vi "Conv2D(CuLab).vi"() -> ()   [LabVIEW 2020]
uses:
  07a04de9-0afa-4073-98d7-d7a9b3666a97.vi
  85e02f6e-3771-4ab4-8b07-b5403419ee50.vi
  <vilib>/Analysis/baseanly.llb/Mean (DBL).vi
  <vilib>/Utility/High Resolution Relative Seconds.vi
  <vilib>/Ngene/CuLab - GPU Accelerated Toolkit/Toolkit/Low_Level/Tensor_Classes/T_Children/T2D/T2D_Children/T2D_SGL/Create_Push.vi
  <vilib>/Ngene/CuLab - GPU Accelerated Toolkit/Toolkit/Low_Level/Tensor_Classes/T_Children/T2D/T2D_Children/T2D_SGL/Create.vi
  <vilib>/Ngene/CuLab - GPU Accelerated Toolkit/Toolkit/Low_Level/Tensor_Classes/T_Children/T2D/T2D_Children/T2D_SGL/Push.vi
  <vilib>/Ngene/CuLab - GPU Accelerated Toolkit/Toolkit/API/Signal Processing/Signal Operation/Convolution/T2D/CU_Convolution_T2D_SGL.vi
  <vilib>/Ngene/CuLab - GPU Accelerated Toolkit/Toolkit/Low_Level/Tensor_Classes/T_Children/T2D/T2D_Children/T2D_SGL/Pull.vi
  <vilib>/Utility/file.llb/Write Delimited Spreadsheet (DBL).vi
  <vilib>/Ngene/CuLab - GPU Accelerated Toolkit/Toolkit/CuLab.lvlib
  <vilib>/Analysis/NI_AALBase.lvlib
  <vilib>/Ngene/CuLab - GPU Accelerated Toolkit/Toolkit/Low_Level/Tensor_Classes/T_Children/T2D/T2D_Children/T2D_SGL/T2D_SGL.lvclass
panel:
  out "Results(s)":dbl[][](array[numeric])=[[0.00010705700000002594, 0.00010179500000006669, 8.743699999996579e-05, 0.00013704700000005232, 0.00013673900000000573, 0.0001405470000000264, 9.487500000005866e-05], [0.0002289619999999104, 0.00020736999999996898, 0.0002290920000000085, 0.0002625960000000305, 0.00021987199999998097, 0.00028411300000001914, 0.0002884970000000919], [0.0006495570000001294, 0.0006395609999999863, 0.0006828300000000808, 0.0007422900000000254, 0.000774169000000029, 0.0007969729999999231, 0.0009009919999999739], [0.0024165789999999274, 0.0023316960000001074, 0.002342025000000092, 0.002518009000000063, 0.0027397600000000468, 0.0028357809999999973, 0.003246644000000032], [0.008428050000000268, 0.008873763999999937, 0.00909312199999988, 0.009545339999999953, 0.010620593000000155, 0.011503052999999852, 0.012151290000000188]] format="%.4p"
  in  "algorithm":enum32{"direct", "frequency domain"}(ring)
  out "error out":errorcluster
  in  "Kernel Size":i32[](array[numeric])=[3, 5, 7, 9, 11, 13, 15]
  in  "Image Size":i32[](array[numeric])=[128, 256, 512, 1024, 2048]
  in  "Batch":i32=100
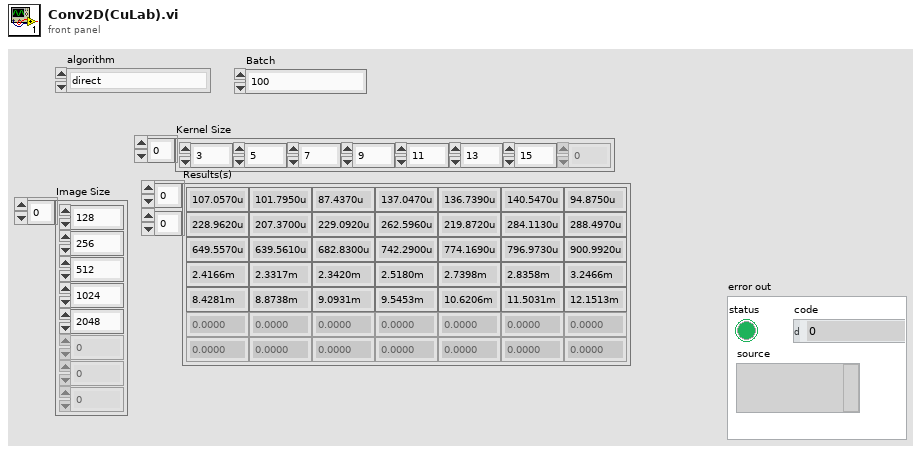
[diagram p1: front panel]
types:
  T1 = typedef "CuLab.lvlib/Properties.ctl" = cluster{"Device ID":i32, "Name":string}
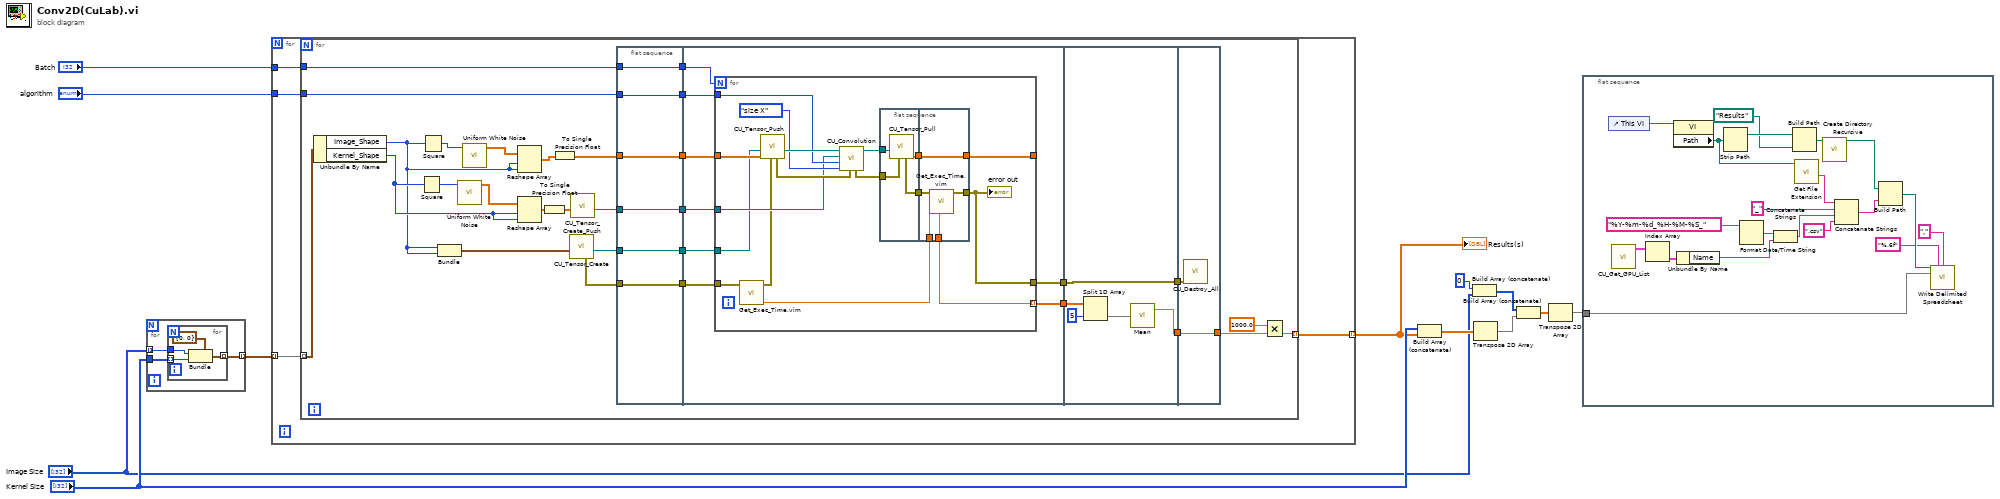
[diagram p0: block diagram]
diagram:
  n1 = for {
    tunnel: "Image Size" -> [w14] mode=indexing
    tunnel: "Kernel Size" -> [w15]
    tunnel: [w13] -> w11 mode=indexing
    n2 = for {
      tunnel: w15 -> [w18] mode=indexing
      tunnel: w14 -> [w19]
      tunnel: [w17] -> w13 mode=indexing
      n3 = Bundle(cluster=cluster{"Image_Shape":i32, "Kernel_Shape":i32} {"Image_Shape"=0, "Kernel_Shape"=0}, "Image_Shape"=w19, "Kernel_Shape"=w18) -> (w17:cluster{"Image_Shape":i32, "Kernel_Shape":i32})
    }
  }
  n4 = for {
    tunnel: w11 -> [w23] mode=indexing
    tunnel: "Batch" -> [w20]
    tunnel: [w22] -> w3 mode=indexing
    tunnel: "algorithm" -> [w21]
    n5 = for {
      tunnel: w23 -> [w48] mode=indexing
      tunnel: [w25] -> w22 mode=indexing
      tunnel: w21 -> [w28]
      tunnel: w20 -> [w27]
      n6 = Unbundle By Name(w48) -> ("Image_Shape"=w39:i32, "Kernel_Shape"=w43:i32)
      n7 = Square(x=w43) -> (x^2=w40:i32)
      n8 = Square(x=w39) -> (x^2=w26:i32)
      n9 = Bundle("Image_Shape"=w39, "Image_Shape"=w39) -> (w53:cluster{"Image_Shape":i32, "Image_Shape":i32})  [unwired: 1 in]
      n10 = call <vilib>:"Uniform White Noise.vi"("samples"=w40) -> ("uniform white noise"=w41:dbl[])  [unwired: 9 in, 1 out]
      n11 = call <vilib>:"Uniform White Noise.vi"("samples"=w26) -> ("uniform white noise"=w42:dbl[])  [unwired: 9 in, 1 out]
      n12 = Reshape Array(w42, w39, w39) -> (w50:dbl[][])
      n13 = Reshape Array(w41, w43, w43) -> (w51:dbl[][])
      n14 = To Single Precision Float(number=w51) -> (single precision float=w33:sgl[][])
      n15 = To Single Precision Float(number=w50) -> (single precision float=w32:sgl[][])
      n16 = call-poly <vilib>:"CU_Tensor_Create.vi"("T2D_Dims"=w53) -> ("T2D_SGL out"=w49:refnum<class "T2D_SGL.lvclass">, "error out"=w52:errorcluster)  [unwired: 9 in]
      n17 = call-poly <vilib>:"CU_Tensor_Create_Push.vi"("CPU_Data_2D_SGL"=w33) -> ("T2D_SGL out"=w44:refnum<class "T2D_SGL.lvclass">)  [unwired: 9 in, 1 out]
      n18 = flat-sequence {
        tunnel: w28 -> [w56]
        tunnel: w52 -> [w55]
        tunnel: w49 -> [w57]
        tunnel: w44 -> [w58]
        tunnel: w32 -> [w59]
        tunnel: [w59] -> w38
        tunnel: [w58] -> w37
        tunnel: [w57] -> w36
        tunnel: [w55] -> w35
        tunnel: [w56] -> w34
        tunnel: [w54] -> w31
        tunnel: w27 -> [w54]
        tunnel: [w64] -> w47
        tunnel: w38 -> [w67]
        tunnel: w37 -> [w66]
        tunnel: w36 -> [w62]
        tunnel: w35 -> [w65]
        tunnel: w34 -> [w63]
        tunnel: w31 -> [w61]
        tunnel: [w60] -> w30
        tunnel: w47 -> [w98]
        tunnel: [w98] -> w45
        tunnel: w30 -> [w97]
        tunnel: [w94] -> w29
        tunnel: [w100] -> w46
        tunnel: w45 -> [w99]
        tunnel: w29 -> [w100]
        frame #0 {
        }
        frame #1 {
          n19 = for {
            N: w61 -> [_]
            tunnel: w67 -> [w75]
            tunnel: w66 -> [w74]
            tunnel: w62 -> [w73]
            tunnel: w65 -> [w84]
            tunnel: [w83] -> w64
            tunnel: w63 -> [w78]
            tunnel: [w77] -> _
            tunnel: [w68] -> w60 mode=indexing
            n20 = call "Get_Exec_Time.vim"("error in (no error)"=w84) -> ("T(n)"=w69:dbl, "error out"=w72:errorcluster)  [unwired: 6 in, 1 out]
            n21 = call-poly <vilib>:"CU_Tensor_Push.vi"("error in (no error)"=w72, "CPU_Data_2D_SGL"=w75, "T2D_SGL in"=w73) -> ("T2D_SGL out"=w81:refnum<class "T2D_SGL.lvclass">, "error out"=w82:errorcluster)  [unwired: 7 in]
            n22 = call-poly <vilib>:"CU_Convolution.vi"("error in"=w82, "output size"=enum32{"full", "size X", "compact"}."size X", "algorithm"=w78, "Y"=w74, "X"=w81) -> ("X * Y"=w76:refnum<class "T2D_SGL.lvclass">, "error out"=w79:errorcluster)  [unwired: 5 in]
            n23 = flat-sequence {
              tunnel: w79 -> [w87]
              tunnel: w76 -> [w85]
              tunnel: [w88] -> w71
              tunnel: [w86] -> w70
              tunnel: [w92] -> w77
              tunnel: [w91] -> w83
              tunnel: w71 -> [w93]
              tunnel: w70 -> [w92]
              tunnel: w69 -> [w90]
              tunnel: [w89] -> w68
              frame #0 {
                n24 = call-poly <vilib>:"CU_Tensor_Pull.vi"("error in (no error)"=w87, "T2D_SGL in"=w85) -> ("2D_SGL_Data"=w86:sgl[][], "error out"=w88:errorcluster)  [unwired: 7 in, 1 out]
              }
              frame #1 {
                n25 = call "Get_Exec_Time.vim"("T(n-1)"=w90, "error in (no error)"=w93) -> ("error out"=w91:errorcluster, "dT"=w89:dbl)  [unwired: 5 in, 1 out]
              }
            }
            "error out" <- w83
          }
        }
        frame #2 {
          n26 = Split 1D Array(array=w97, index=5) -> (second subarray=w95:dbl[])  [unwired: 1 out]
          n27 = call-poly <vilib>:"Mean.vi"("X"=w95) -> ("mean"=w94:dbl)  [unwired: 1 out]
        }
        frame #3 {
          n28 = call <vilib>:"CU_Destroy_All.vi"("error in"=w99) -> ()  [unwired: 10 in, 1 out]
        }
      }
      n29 = Multiply(x=1000.0, y=w46) -> (x*y=w25:dbl)
    }
  }
  "Results(s)" <- w3
  n30 = Build Array (concatenate)("Kernel Size", w3) -> (w10:dbl[][])
  n31 = Build Array (concatenate)(0 ("element"), "Image Size") -> (w6:i32[])
  n32 = Transpose 2D Array(2D array=w10) -> (transposed array=w8:dbl[][])
  n33 = Build Array (concatenate)(w6, w8) -> (w7:dbl[][])
  n34 = Transpose 2D Array(2D array=w7) -> (transposed array=w1:dbl[][])
  n35 = flat-sequence {
    tunnel: w1 -> [w120]
    frame #0 {
      n36 = control-ref of="This VI"() -> (w113:refnum<vi>)
      n37 = call <vilib>:"CU_Get_GPU_List.vi"() -> ("Devices"=w104:T1[])  [unwired: 10 in, 1 out]
      n38 = Index Array(array=w104) -> (element=w103:T1)  [unwired: 1 in]
      n39 = property class="VI"(reference=w113) -> ("Path"=w108:path)  [unwired: 1 in, 2 out]
      n40 = Unbundle By Name(w103) -> ("Name"=w101:string)
      n41 = Strip Path(path=w108) -> (stripped path=w112:path)  [unwired: 1 out]
      n42 = Format Date/Time String(time format string (%c)="%Y-%m-%d_%H-%M-%S_") -> (date/time string=w115:string)  [unwired: 2 in]
      n43 = Concatenate Strings(w115, w101) -> (w102:string)
      n44 = Build Path(base path=w112, name or relative path=path "Results") -> (appended path=w111:path)
      n45 = call <vilib>:"Get File Extension.vi"("file"=w108) -> ("filename without extension"=w107:string)  [unwired: 6 in, 4 out]
      n46 = call <vilib>:"Create Directory Recursive.vi"("directory"=w111) -> ("directory copy"=w109:path)  [unwired: 4 in, 2 out]
      n47 = Concatenate Strings(w107, "_" ("string"), w102, ".csv" ("string")) -> (w117:string)
      n48 = Build Path(base path=w109, name or relative path=w117) -> (appended path=w118:path)
      n49 = call-poly <vilib>:"Write Delimited Spreadsheet.vi"("file path (dialog if empty)"=w118, "format (%.3f)"="%.6f", "2D data"=w120, "delimiter (\\t)"="," ("delimiter (\\t)")) -> ()  [unwired: 10 in, 2 out]
    }
  }
